vi "Resample Image.vi"(6 "Decimation":i32=3, 11 "Picture":picture) -> (3 "image data":T1)   [LabVIEW 2024]
uses:
  <vilib>/picture/picture.llb/imagedata.ctl
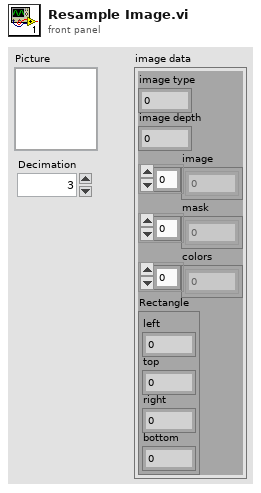
[diagram p1: front panel]
types:
  T1 = typedef "imagedata.ctl" = cluster{"image type":i32, "image depth":i32, "image":u8[], "mask":u8[], "colors":u32[], "Rectangle":cluster{"left":i16, "top":i16, "right":i16, "bottom":i16}}
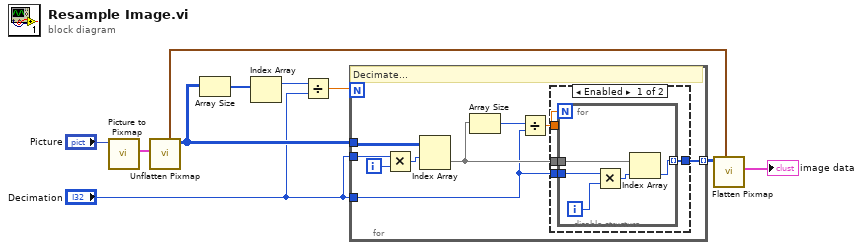
[diagram p0: block diagram]
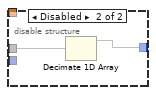
[diagram p2: hidden frame]
diagram:
  n1 = call <vilib>:"Picture to Pixmap.vi"("picture"="Picture") -> ("image data"=w9:T1)  [unwired: 9 in, 1 out]
  n2 = call <vilib>:"Unflatten Pixmap.vi"("image data"=w9) -> ("24-bit pixmap"=w7:u32[][], "top left"=w8:cluster{"x":i16, "y":i16})  [unwired: 4 in, 5 out]
  n3 = Array Size(array=w7) -> (size(s)=w6:i32[])
  n4 = Index Array(array=w6) -> (element=w5:i32)  [unwired: 1 in]
  n5 = Divide(x=w5, y="Decimation") -> (x/y=w4:dbl)
  n6 = for {
    N: w4 -> [_]
    tunnel: w7 -> [w19]
    tunnel: "Decimation" -> [w17]
    tunnel: [w12] -> w3 mode=indexing
    tunnel: "Decimation" -> [w11]
    i -> [w18]
    # "Decimate..."
    n7 = Multiply(x=w17, y=w18) -> (x*y=w16:i32)
    n8 = Index Array(array=w19, index (row)=w16) -> (element=w14:u32[])  [unwired: 1 in]
    n9 = Array Size(array=w14) -> (size(s)=w15:i32)
    n10 = Divide(x=w15, y=w11) -> (x/y=w13:dbl)
    n11 = disable-structure shown="Enabled" {
      disable-tunnel: w14 -> [w23 w30]
      disable-tunnel: w13 -> [w22 _]
      disable-tunnel: [w21 w29] -> w12
      disable-tunnel: w11 -> [w20 _]
      frame Enabled {
        n12 = for {
          N: w22 -> [_]
          tunnel: w23 -> [w27]
          tunnel: [w26] -> w21 mode=indexing
          tunnel: w20 -> [w24]
          i -> [w25]
          n13 = Multiply(x=w24, y=w25) -> (x*y=w28:i32)
          n14 = Index Array(array=w27, index=w28) -> (element=w26:u32)
        }
      }
      frame Disabled {
        n15 = Decimate 1D Array(w30) -> (w29:u32[])  [unwired: 2 out]
      }
    }
  }
  n16 = call <vilib>:"Flatten Pixmap.vi"("top left"=w8, "24-bit pixmap"=w3) -> ("image data"=→"image data":T1)  [unwired: 9 in]
